vi "Initialize_MacroGUI_MD.vi"(8 "Error In":errorcluster, 11 "UI control refnums":T1) -> (0 "Error Out":errorcluster, 2 "Macro Error OUT":bool, 3 "New Index OUT":i32)   [LabVIEW 2012]
doc: "SciScan 1.2 160622"
uses:
  Custom Controls and Typedefs/Macro_MD_UI Control Refnums.ctl
  Custom Controls and Typedefs/Delete Button.ctl
  Custom Controls and Typedefs/Edit Button.ctl
  Custom Controls and Typedefs/Timing Estimate Cluster.ctl
  CommonResource VIs/Timing/Timing Indicator.ctl
  Custom Controls and Typedefs/Load from PSM Button.ctl
  FGV_MacroCore_Commands.ctl
  CommonResource VIs/UI Control and Indicator properties_Commands.ctl
  MacroFileIO_Commands.ctl
  CommonResource VIs/Enable-Disable SCISCAN controls_Command.ctl
  <vilib>/Utility/miscctls.llb/LVRowAndColumnUnsignedTypeDef.ctl
  <vilib>/Utility/miscctls.llb/LVRowAndColumnTypeDef.ctl
  SCISCAN Image display to Enum_Commands.ctl
panel:
  # "(hh:mm:ss)"
  # "(hh:mm:ss)"
  # "(hh:mm:ss)"
  # "(hh:mm:ss)"
  # "(hh:mm:ss)"
  # "(hh:mm:ss)"
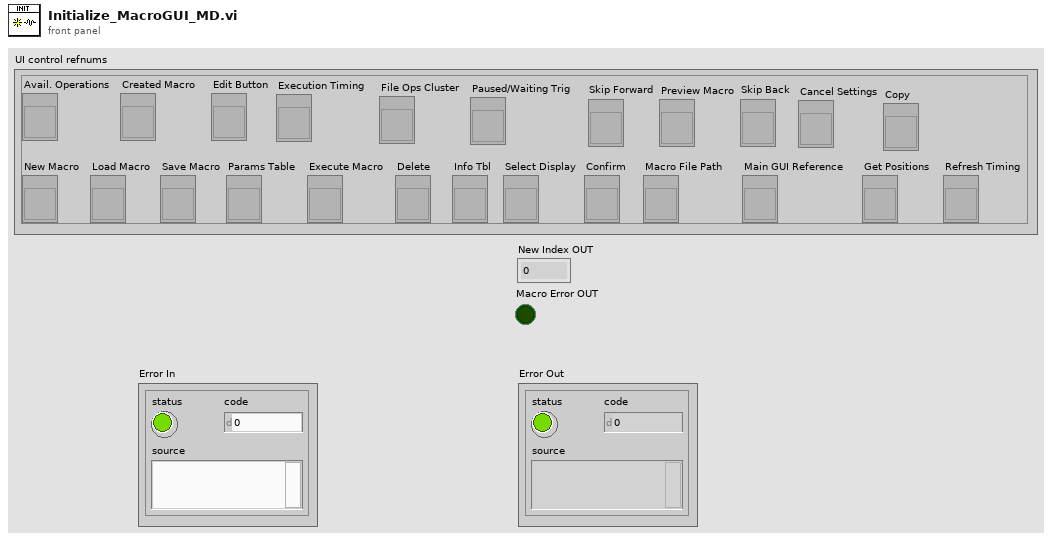
[diagram p1: front panel]
types:
  T1 = typedef "Macro_MD_UI Control Refnums.ctl" = cluster{"Avail. Operations":refnum<vi>, "Created Macro":refnum<vi>, "Load Macro":refnum<vi>, "Save Macro":refnum<vi>, "Params Table":refnum<vi>, "Delete":refnum<vi>, "Edit Button":refnum<vi>, "Execute Macro":refnum<vi>, "Info Tbl":refnum<vi>, "Execution Timing":refnum<vi>, "Select Display":refnum<vi>, "File Ops Cluster":refnum<vi>, "Paused/Waiting Trig":refnum<vi>, "Confirm":refnum<vi>, "New Macro":refnum<vi>, "Preview Macro":refnum<vi>, "Skip Forward":refnum<vi>, "Skip Back":refnum<vi>, "Macro File Path":refnum<vi>, "Main GUI Reference":refnum<vi>, "Cancel Settings":refnum<vi>, "Get Positions":refnum<vi>, "Copy":refnum<vi>, "Refresh Timing":refnum<vi>}
  T2 = enum32{"None", "LabVIEW", "Mac OS", "Windows", "Default"}
  T3 = typedef "UI Control and Indicator properties_Commands.ctl" = enum16{"Enable", "Disable", "Disable and Grey", "Make Visible", "Make Invisible"}
  T4 = typedef "Enable-Disable SCISCAN controls_Command.ctl" = enum16{"Enable the items disabled earlier", "Disable", "Disable and Gray", "Enable all (except those in skip list)"}
  T5 = typedef "MacroFileIO_Commands.ctl" = enum16{"Get Macro Info", "Initialize", "New Macro", "Load Macro", "Save", "Save in today's folder", "Update Settings File", "Add Settings File", "Delete Settings File", "Update Macro Text", "Save As", "Read Temp File"}
  T6 = enum8{"Enabled", "Disabled", "Disabled and Grayed Out"}
  T7 = typedef "FGV_MacroCore_Commands.ctl" = enum16{"Initialize", "Get Array", "Load macro from file", "Insert Item", "Insert at End", "Edit Parameter String", "Delete instruction", "Move Items", "Save", "SaveAs", "UpdateInfoTable", "Edit Settings File", "New Macro", "Read Temp File", "Delete Multiple"}
  T8 = typedef "LVRowAndColumnUnsignedTypeDef.ctl" = cluster{"Row":u32, "Column":u32}
  T9 = typedef "LVRowAndColumnTypeDef.ctl" = cluster{"Row":i32, "Column":i32}
  T10 = typedef "SCISCAN Image display to Enum_Commands.ctl" = enum16{"Initialize", "SCISCAN disp to Enum", "Enum to SCISCAN disp"}
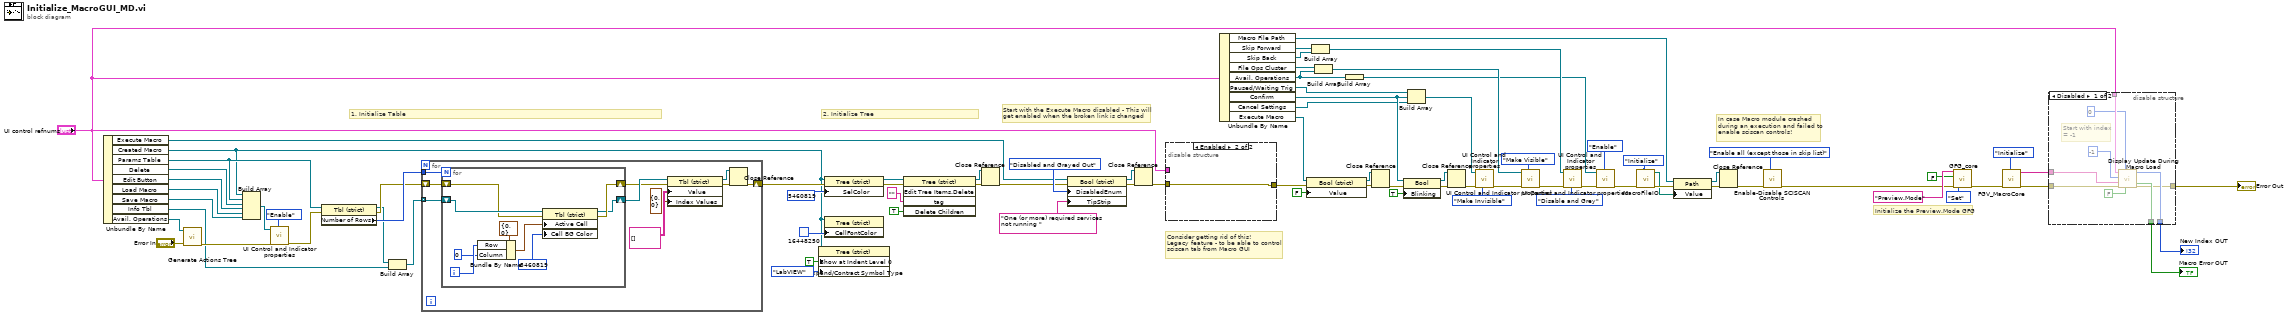
[diagram p0: block diagram]
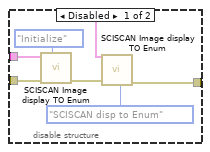
[diagram p2: hidden frame]
diagram:
  # "Consider getting rid of this!\nLegacy feature - to be able to control \nsciscan tab from Macro GUI"
  # "Initialize the Preview.Mode GFG"
  # "In case Macro module crashed\nduring an execution and failed to\nenable sciscan controls!"
  # "Start with the Execute Macro disabled - This will\nget enabled when the broken link is changed"
  # "2. Initialize Tree"
  # "1. Initialize Table"
  n1 = Unbundle By Name("UI control refnums") -> ("Execute Macro"=w67:refnum<vi>, "Created Macro"=w3:refnum<vi>, "Params Table"=w6:refnum<vi>, "Delete"=w66:refnum<vi>, "Edit Button"=w65:refnum<vi>, "Load Macro"=w64:refnum<vi>, "Save Macro"=w63:refnum<vi>, "Info Tbl"=w7:refnum<vi>, "Avail. Operations"=w16:refnum<vi>)
  n2 = call "Generate Actions Tree.vi"("error in (no error)"="Error In", "Tree Refnum IN"=w16) -> ("error out"=w14:errorcluster)  [unwired: 9 in]
  n3 = Build Array(w3, w6, w66, w65, w64, w63) -> (w62:refnum<vi>[])
  n4 = call "UI Control and Indicator properties.vi"("Enable Command"=UI_Control_and_Indicator_properties_Commands."Enable", "Error In"=w14, "Control Refnums"=w62) -> ("Error Out"=w61:errorcluster)  [unwired: 8 in]
  n5 = property class="Tbl (strict)"(reference=w6, error in=w61) -> (reference out=w5:refnum<vi>, error out=w83:errorcluster, "Number of Rows"=w84:u32)
  n6 = Build Array(w5, w7) -> (w4:refnum<vi>[])
  n7 = for {
    tunnel: w84 -> [w94]
    tunnel: w4 -> [w85] mode=indexing
    shift-right: [w88] -> w75
    shift-left: w83 -> [w93]
    n8 = for {
      N: w94 -> [_]
      shift-right: [w96] -> w89
      shift-left: w93 -> [w99]
      shift-right: [w95] -> w90
      shift-left: w85 -> [w100]
      i -> [w102]
      n9 = Bundle By Name(cluster=T9 {"Row"=0, "Column"=0} ("Active Cell:Active Cell"), "Row"=w102, "Column"=0) -> (w98:T9)
      n10 = property class="Tbl (strict)"(reference=w100, error in=w99, "Active Cell"=w98, "Cell BG Color"=u32 5460819 ("Active Cell:Cell Background Color")) -> (reference out=w95:refnum<vi>, error out=w96:errorcluster)
    }
    n11 = property class="Tbl (strict)"(reference=w90, error in=w89, "Value"=string[][] [], "Index Values"=T8 {"Row"=0, "Column"=0}) -> (reference out=w92:refnum<vi>, error out=w91:errorcluster)
    n12 = Close Reference(reference=w92, error in (no error)=w91) -> (error out=w88:errorcluster)
  }
  n13 = property class="Tree (strict)"(reference=w3, "Show at Indent Level 0"=TRUE ("Expand/Contract Symbol:Show Symbol at Root"), "Expand/Contract Symbol Type"=T2."LabVIEW" ("Expand/Contract Symbol:Symbol Type")) -> ()  [unwired: 1 in, 2 out]
  n14 = property class="Tree (strict)"(reference=w3, error in=w75, "SelColor"=u32 5460819 ("Active Cell:Cell Background Color")) -> (reference out=w79:refnum<vi>, error out=w80:errorcluster)
  n15 = property class="Tree (strict)"(reference=w3, "CellFontColor"=u32 16448250) -> ()  [unwired: 1 in, 2 out]
  n16 = invoke class="Tree (strict)" method="Edit Tree Items.Delete"(reference=w79, error in=w80, "tag"="" ("Tag"), "Delete Children"=TRUE ("Delete Children?")) -> (reference out=w77:refnum<vi>, error out=w78:errorcluster)  [unwired: 1 in, 3 out]
  n17 = Close Reference(reference=w77, error in (no error)=w78) -> (error out=w20:errorcluster)
  n18 = property class="Bool (strict)"(reference=w67, error in=w20, "DisabledEnum"=T6."Disabled and Grayed Out" ("Disabled"), "TipStrip"="One (or more) required services not running " ("Tip Strip")) -> (reference out=w71:refnum<vi>, error out=w72:errorcluster)
  n19 = Close Reference(reference=w71, error in (no error)=w72) -> (error out=w60:errorcluster)
  n20 = disable-structure shown="Enabled" {
    disable-tunnel: w60 -> [w106 w110]
    disable-tunnel: [w105 w110] -> w59
    disable-tunnel: "UI control refnums" -> [w104 _]
    frame Disabled {
      n21 = call "SCISCAN Image display TO Enum .vi"("SCISCAN Image display_to_Enum_Commands"=SCISCAN_Image_display_to_Enum_Commands."Initialize", "Error In"=w106, "UI control refnums"=w104) -> ("Error Out"=w107:errorcluster)  [unwired: 8 in]
      n22 = call "SCISCAN Image display TO Enum .vi"("SCISCAN Image display_to_Enum_Commands"=SCISCAN_Image_display_to_Enum_Commands."SCISCAN disp to Enum", "Error In"=w107, "UI control refnums"=w104) -> ("Error Out"=w105:errorcluster)  [unwired: 8 in]
    }
    frame Enabled {
    }
  }
  n23 = Unbundle By Name("UI control refnums") -> ("Macro File Path"=w35:refnum<vi>, "Skip Forward"=w39:refnum<vi>, "Skip Back"=w38:refnum<vi>, "File Ops Cluster"=w51:refnum<vi>, "Avail. Operations"=w12:refnum<vi>, "Paused/Waiting Trig"=w54:refnum<vi>, "Confirm"=w46:refnum<vi>, "Cancel Settings"=w17:refnum<vi>, "Execute Macro"=w48:refnum<vi>)
  n24 = property class="Bool (strict)"(reference=w48, error in=w59, "Value"=FALSE) -> (reference out=w56:refnum<vi>, error out=w57:errorcluster)
  n25 = Build Array(w39, w38) -> (w37:refnum<vi>[])
  n26 = Build Array(w51, w12) -> (w49:refnum<vi>[])
  n27 = Build Array(w12) -> (w10:refnum<vi>[])
  n28 = Close Reference(reference=w56, error in (no error)=w57) -> (error out=w47:errorcluster)
  n29 = property class="Bool"(reference=w46, error in=w47, "Blinking"=TRUE) -> (reference out=w43:refnum<vi>, error out=w44:errorcluster)
  n30 = Build Array(w54, w46, w17) -> (w53:refnum<vi>[])
  n31 = Close Reference(reference=w43, error in (no error)=w44) -> (error out=w42:errorcluster)
  n32 = call "UI Control and Indicator properties.vi"("Enable Command"=UI_Control_and_Indicator_properties_Commands."Make Invisible", "Error In"=w42, "Control Refnums"=w53) -> ("Error Out"=w50:errorcluster)  [unwired: 8 in]
  n33 = call "UI Control and Indicator properties.vi"("Enable Command"=UI_Control_and_Indicator_properties_Commands."Make Visible", "Error In"=w50, "Control Refnums"=w49) -> ("Error Out"=w41:errorcluster)  [unwired: 8 in]
  n34 = call "UI Control and Indicator properties.vi"("Enable Command"=UI_Control_and_Indicator_properties_Commands."Disable and Grey", "Error In"=w41, "Control Refnums"=w37) -> ("Error Out"=w13:errorcluster)  [unwired: 8 in]
  n35 = call "UI Control and Indicator properties.vi"("Enable Command"=UI_Control_and_Indicator_properties_Commands."Enable", "Error In"=w13, "Control Refnums"=w10) -> ("Error Out"=w9:errorcluster)  [unwired: 8 in]
  n36 = call "MacroFileIO.vi"("MacroFileIO_Command"=MacroFileIO_Commands."Initialize" ("FGV_MacroFileIO_Command"), "Error In"=w9) -> ("Macro File Path OUT"=w31:path, "Error Out"=w34:errorcluster)  [unwired: 8 in, 4 out]
  n37 = property class="Path"(reference=w35, error in=w34, "Value"=w31) -> (reference out=w32:refnum<vi>, error out=w33:errorcluster)
  n38 = Close Reference(reference=w32, error in (no error)=w33) -> (error out=w29:errorcluster)
  n39 = call "Enable-Disable SCISCAN Controls.vi"("Enable-Disable SCISCAN Controls_Command"=Enable-Disable_SCISCAN_controls_Command."Enable all (except those in skip list)", "Error In"=w29) -> ("Error Out"=w8:errorcluster)  [unwired: 9 in]
  n40 = call "GFG_core.vi"("Variable Name in"="Preview.Mode", "Variant in"=FALSE, "error in (no error)"=w8, "Action"=enum16{"Init", "Set", "Get", "Clear"}."Set") -> ("error out"=w19:errorcluster)  [unwired: 9 in, 6 out]
  n41 = call "FGV_MacroCore.vi"("MacroFGV_Commands"=FGV_MacroCore_Commands."Initialize", "Error In"=w19) -> ("Error Out"=w25:errorcluster, "Macro String Array"=w23:string[])  [unwired: 5 in, 3 out]
  n42 = disable-structure shown="Disabled" {
    disable-tunnel: w25 -> [w119 w120]
    disable-tunnel: "UI control refnums" -> [w118 _]
    disable-tunnel: w23 -> [w117 _]
    disable-tunnel: [w114 _] -> w22
    disable-tunnel: [w113 _] -> w21
    disable-tunnel: [w112 w120] -> w18
    frame Disabled {
      # "Start with index\n= -1"
      n43 = call "Display Update During Macro Load.vi"("Macro Error IN"=FALSE, "New Index IN"=0, "error in (no error)"=w119, "Macro Array IN"=w117, "Previous Index IN"=-1, "UI control refnums"=w118) -> ("error out"=w112:errorcluster, "New Index OUT"=w113:i32, "Macro Error OUT"=w114:bool)  [unwired: 3 in]
    }
    frame Enabled {
    }
  }
  "Error Out" <- w18
  "Macro Error OUT" <- w22
  "New Index OUT" <- w21
